vi "Test - AI.vi"() -> ()   [LabVIEW 2020]
uses:
  <vilib>/Utility/error.llb/Error Cluster From Error Code.vi
  <vilib>/myRIO/Common/Instrument Driver Framework/myRIO v1.0/AI/vis/myRIO v1.0 Read AI.vi
  <vilib>/myRIO/Instrument Drivers/Onboard IO/AI/AI.lvlib
panel:
  in  "Stop":bool
  out "Battery Voltage (B/AI2 (Pin 7)) 2":dbl
  out "Solar Voltage  (B/AI1 (Pin 5)) 2":dbl
  out "Battery Current (B/AI0 (Pin 3)) 2":dbl
  out "Solar Current (A/AI3 (Pin 9)) 2":dbl
  out "Temp 3 (A/AI2 (Pin 7)) 2":dbl
  out "Temp 2 (A/AI1 (Pin 5)) 2":dbl
  out "Temp 1 (A/AI0 (Pin 3)) 2":dbl
  out "Error Out":errorcluster
  in  "Error In":errorcluster
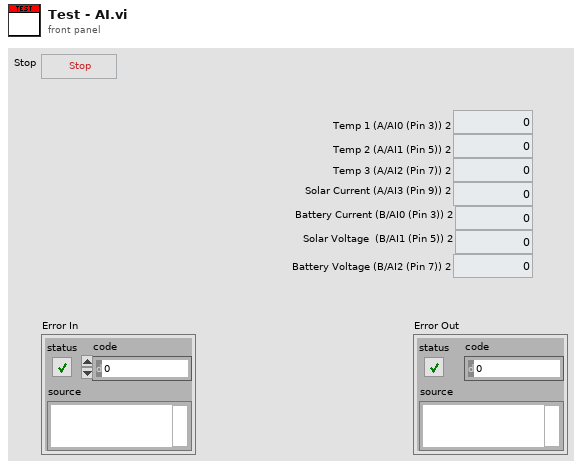
[diagram p1: front panel]
types:
  T1 = typedef "AI.lvlib/AI Reference.ctl" = cluster{"myRIO Reference":T2, "AI Channels List":T6, "AI Scaling Constants List":T8}
  T2 = typedef "myRIO Generic Hardware Reference.ctl" = cluster{"myRIO Model":T3, "myRIO Hardware Reference":T4}
  T3 = typedef "Hardware Version Enum.ctl" = enum16{"Unknown", "myRIO-1900", "myRIO-1950", "roboRIO", "NI ELVIS RIO CM", "ELVIS III"}
  T4 = typedef "myRIO v1.0 Reference.ctl" = cluster{"Generic FPGA Reference":T5, "Allow multiple opens":bool}
  T5 = typedef "Generic FPGA Reference.ctl" = refnum<k20>
  T6 = typedef "AI Channels List.ctl" = T7[]
  T7 = typedef "AI Channels Enum.ctl" = enum16{"Not Connected", "AudioIn/Left", "AudioIn/Right", "C/AI0", "C/AI1", "A/AI0", "A/AI1", "A/AI2", "A/AI3", "A/AI4", "A/AI5", "A/AI6", "A/AI7", "B/AI0", "B/AI1", "B/AI2", "B/AI3", "B/AI4", "B/AI5", "B/AI6", "B/AI7", "AI/AI0", "AI/AI1", "AI/AI2", "AI/AI3", "A/AI0 (DIFF)", "A/AI1 (DIFF)", "A/AI2 (DIFF)", "A/AI3 (DIFF)", "B/AI0 (DIFF)", "B/AI1 (DIFF)", "B/AI2 (DIFF)", "B/AI3 (DIFF)"}
  T8 = typedef "Analog Scaling Constants List.ctl" = T9[]
  T9 = typedef "Analog Scaling Constants.ctl" = cluster{"LSB Weight (Volts)":dbl, "Offset (Volts)":dbl, "Signed?":bool}
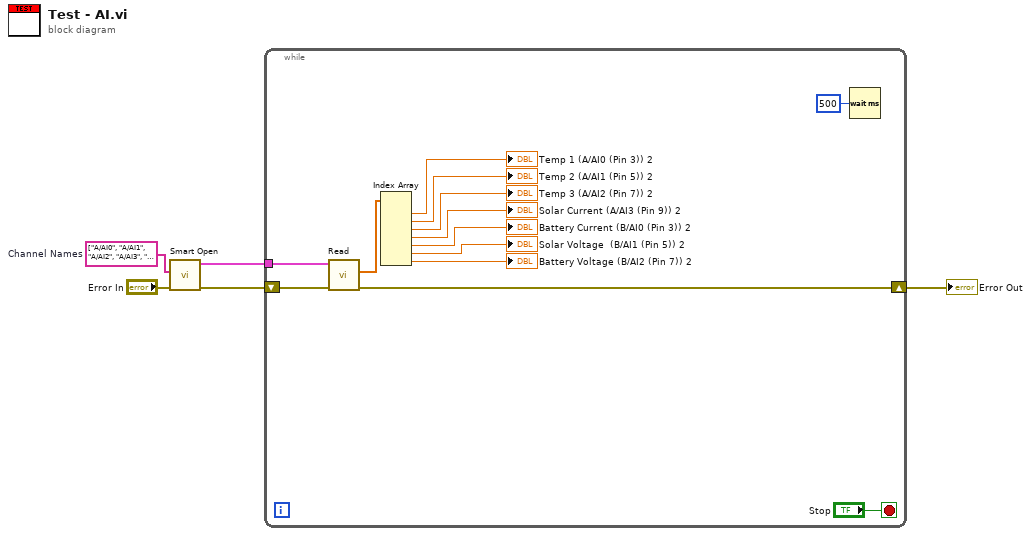
[diagram p0: block diagram]
diagram:
  w2 = tag[] ["A/AI0", "A/AI1", "A/AI2", "A/AI3", "B/AI0", "B/AI1", "B/AI2"]  # Channel Names
  n1 = call <vilib>:"Smart Open.vi"("error in (no error)"="Error In", "Channel Names"=w2) -> ("error out"=w4:errorcluster, "AI Ref Out"=w1:T1)  [unwired: 8 in]
  n2 = while {
    tunnel: w1 -> [w15]
    shift-right: [w17] -> w3
    shift-left: w4 -> [w18]
    stop <- "Stop" stop-if-true
    n3 = call <vilib>:"Read.vi"("error in (no error)"=w18, "AI Ref In"=w15) -> ("error out"=w17:errorcluster, "Values"=w16:dbl[])  [unwired: 7 in, 1 out]
    n4 = Index Array(array=w16) -> (element #1=→"Temp 1 (A/AI0 (Pin 3)) 2":dbl, element #2=→"Temp 2 (A/AI1 (Pin 5)) 2":dbl, element #3=→"Temp 3 (A/AI2 (Pin 7)) 2":dbl, element #4=→"Solar Current (A/AI3 (Pin 9)) 2":dbl, element #5=→"Battery Current (B/AI0 (Pin 3)) 2":dbl, element #6=→"Solar Voltage  (B/AI1 (Pin 5)) 2":dbl, element #7=→"Battery Voltage (B/AI2 (Pin 7)) 2":dbl)  [unwired: 7 in]
    n5 = Wait (ms)(milliseconds to wait=u32 500) -> ()  [unwired: 1 out]
  }
  "Error Out" <- w3
